vi "I2C Write To Lights.vi"   [LabVIEW 2014]
uses:
  Robot Global Data.vi
types:
  T1 = typedef "Elevator Status.ctl" = cluster{"State":T2, "Eject Piston":bool, "Height":dbl, "Top Limit Switch":bool, "Bottom Limit Switch":bool, "Target":dbl, "In Range":bool, "Enc Value":dbl, "Limit Override":bool, "Mode":T3, "Stabilizer":bool, "Finger":bool, "Low IR":bool, "High IR":bool, "Motor Out":dbl}
  T2 = typedef "Elevator State.ctl" = enum16{"Idle", "Goto Load Position", "Wait for Load", "Load Drop", "Load Lift", "Drop Stack", "Goto Eject Position", "Eject "}
  T3 = typedef "Elevator Mode.ctl" = enum16{"Manual", "Safe", "Auto"}
  T4 = typedef "WPI_DriverStationRobotMode2.ctl" = enum16{"Autonomous Disabled", "Autonomous Enabled", "Teleop Disabled", "Teleop Enabled", "Disconnected", "Finish", "Test Disabled", "Test Enabled", "Emergency Stopped"}
  T5 = typedef "WPI_I2CDevRef.ctl" = cluster{"DevStatus":errorcluster, "Controller":T6, "Device Address":u8, "Handle":i32, "I2C Bus":T7}
  T6 = typedef "FPGA_TypedefDigitalModule.ctl" = enum16{"Controller 1"}
  T7 = typedef "i2c_bus.ctl" = enum16{"I2C On-Board", "I2C MXP", "Invalid"}
  T8 = typedef "WPI_DriverStationAllianceInfo.ctl" = enum16{"Red", "Blue", "Invalid"}
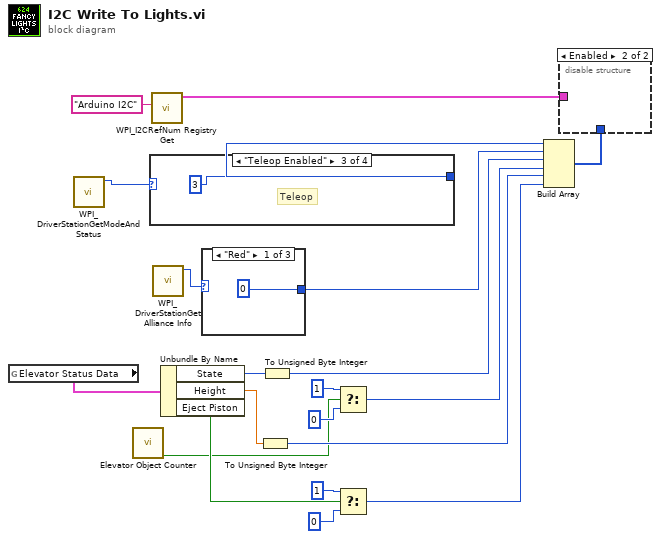
[diagram p0: block diagram]
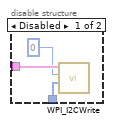
[diagram p2: hidden frame]
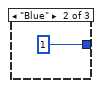
[diagram p3: hidden frame]
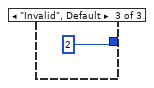
[diagram p4: hidden frame]
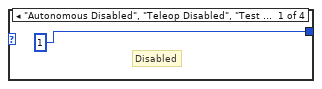
[diagram p5: hidden frame]
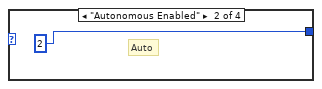
[diagram p6: hidden frame]
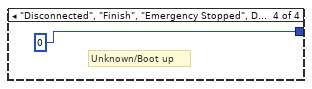
[diagram p7: hidden frame]
diagram:
  n1 = global read "Robot Global Data.vi" "Elevator Status Data"() -> (w13:T1)
  n2 = call <vilib>:"WPI_DriverStationGetModeAndStatus.vi"() -> ("Robot Mode"=w18:T4)  [unwired: 10 in, 1 out]
  n3 = call "Elevator Object Counter.vi"() -> ("Have Trashcan"=w1:bool)  [unwired: 10 in, 1 out]
  n4 = case shown="\"Teleop Enabled\"" w18 {
    tunnel: [u8 1 ("I2CRegister") u8 2 ("I2CRegister") u8 3 ("I2CRegister") u8 0 ("I2CRegister")] -> w17
    frame "Autonomous Disabled", "Teleop Disabled", "Test Disabled" {
      # "Disabled"
    }
    frame "Autonomous Enabled" {
      # "Auto"
    }
    frame "Teleop Enabled" {
      # "Teleop"
    }
    frame "Disconnected", "Finish", "Emergency Stopped", Default {
      # "Unknown/Boot up"
    }
  }
  n5 = call <vilib>:"WPI_I2CRefNum Registry Get.vi"("refnum name"="Arduino I2C") -> ("I2CDevRef"=w20:T5)  [unwired: 9 in, 1 out]
  n6 = call <vilib>:"WPI_DriverStationGet Alliance Info.vi"() -> ("Alliance"=w16:T8)  [unwired: 10 in, 1 out]
  n7 = Unbundle By Name(w13) -> ("State"=w12:T2, "Height"=w7:dbl, "Eject Piston"=w3:bool)
  n8 = case shown="\"Red\"" w16 {
    tunnel: [u8 0 u8 1 u8 2 ("I2CRegister")] -> w15
    frame "Red" {
    }
    frame "Blue" {
    }
    frame "Invalid", Default {
    }
  }
  n9 = To Unsigned Byte Integer(number=w7) -> (unsigned 8bit integer=w6:u8)
  n10 = To Unsigned Byte Integer(number=w12) -> (unsigned 8bit integer=w11:u8)
  n11 = Select(t=u8 1 ("unsigned 8bit integer"), s=w1, f=u8 0 ("unsigned 8bit integer")) -> (s? t:f=w8:u8)
  n12 = Select(t=u8 1 ("unsigned 8bit integer"), s=w3, f=u8 0 ("unsigned 8bit integer")) -> (s? t:f=w2:u8)
  n13 = Build Array(w17, w15, w11, w8, w6, w2) -> (w14:u8[])
  n14 = disable-structure shown="Enabled" {
    disable-tunnel: w20 -> [w30 _]
    disable-tunnel: w14 -> [w28 _]
    frame Disabled {
      n15 = call <vilib>:"WPI_I2CWrite.vi"("I2CDataToSend"=w28, "I2CRegister"=u8 0, "I2CDevRef"=w30) -> ()  [unwired: 7 in, 2 out]
    }
    frame Enabled {
    }
  }
